vi "svx_Autoscale Y.vi"(9 "Cropped Info":cluster{"First Index":i32, "Length":i32}, 11 "Plots":cluster{"x0":dbl, "dx":dbl, "Y":dbl[]}[](array[cluster])) -> (1 "min":dbl, 3 "max":dbl)   [LabVIEW 2017, in "SVX Waterfall Graph.xctl"]
uses:
  <vilib>/addons/_XControls/Waterfall Graph/SVX Waterfall Graph.xctl
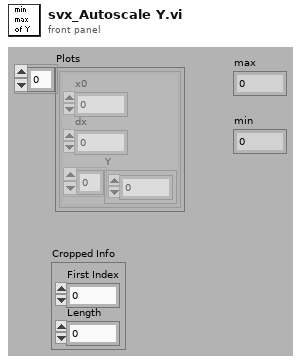
[diagram p1: front panel]
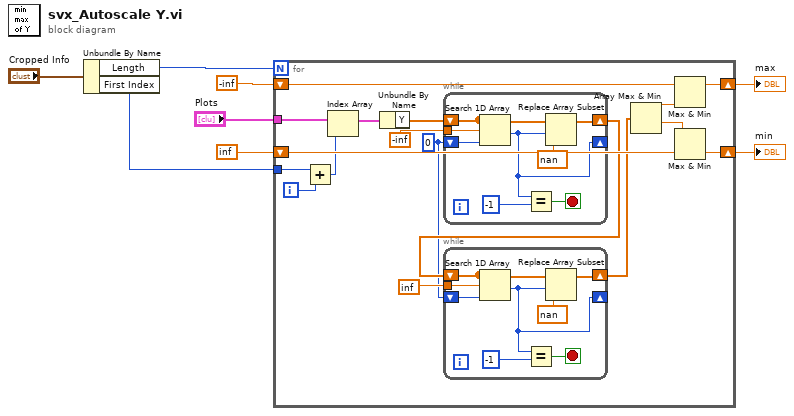
[diagram p0: block diagram]
diagram:
  n1 = Unbundle By Name("Cropped Info") -> ("Length"=w3:i32, "First Index"=w1:i32)
  n2 = for {
    N: w3 -> [_]
    shift-right: [w20] -> w7
    shift-left: -inf -> [w25]
    shift-right: [w21] -> w8
    shift-left: inf -> [w22]
    tunnel: "Plots" -> [w17]
    tunnel: w1 -> [w15]
    i -> [w16]
    w9 = 0 ("index of element")
    n3 = Add(x=w15, y=w16) -> (x+y=w14:i32)
    n4 = Index Array(array=w17, index=w14) -> (element=w13:cluster{"x0":dbl, "dx":dbl, "Y":dbl[]})
    n5 = Unbundle By Name(w13) -> ("Y"=w18:dbl[])
    n6 = while {
      tunnel: -inf -> [w41]
      shift-right: [w34] -> _
      shift-left: w9 -> [w38]
      shift-right: [w36] -> w12
      shift-left: w18 -> [w37]
      stop <- w40 stop-if-true
      n7 = Search 1D Array(1D array=w37, element=w41, start index (0)=w38) -> (index of element=w34:i32)
      n8 = Equal?(x=w34, y=-1) -> (x = y?=w40:bool)
      n9 = Replace Array Subset(array=w37, new element=nan ("new element/subarray"), index=w34) -> (w36:dbl[])
    }
    n10 = while {
      tunnel: inf -> [w33]
      shift-right: [w26] -> _
      shift-left: w9 -> [w30]
      shift-right: [w28] -> w11
      shift-left: w12 -> [w29]
      stop <- w32 stop-if-true
      n11 = Search 1D Array(1D array=w29, element=w33, start index (0)=w30) -> (index of element=w26:i32)
      n12 = Equal?(x=w26, y=-1) -> (x = y?=w32:bool)
      n13 = Replace Array Subset(array=w29, new element=nan ("new element/subarray"), index=w26) -> (w28:dbl[])
    }
    n14 = Array Max & Min(array=w11) -> (max value=w24:dbl, min value=w23:dbl)  [unwired: 2 out]
    n15 = Max & Min(x=w25, y=w24) -> (max(x,y)=w20:dbl)  [unwired: 1 out]
    n16 = Max & Min(x=w23, y=w22) -> (min(x,y)=w21:dbl)  [unwired: 1 out]
  }
  "min" <- w8
  "max" <- w7
